vi "blokada wysylania manipulatora.vi"(6 "Y":i32, 8 "Zaxis":i32, 9 "X axis":i32, 10 "wysylanie":bool) -> (0 "zakres Z":bool, 1 "zakres X":bool, 2 "blokadaa":bool, 3 "Wyslij":bool, 4 "zakres Y":bool)   [LabVIEW 2015]
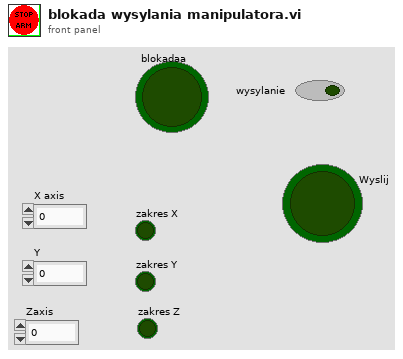
[diagram p1: front panel]
types:
  T1 = enum16{"Rising Edge", "Falling Edge", "Any Edge"}
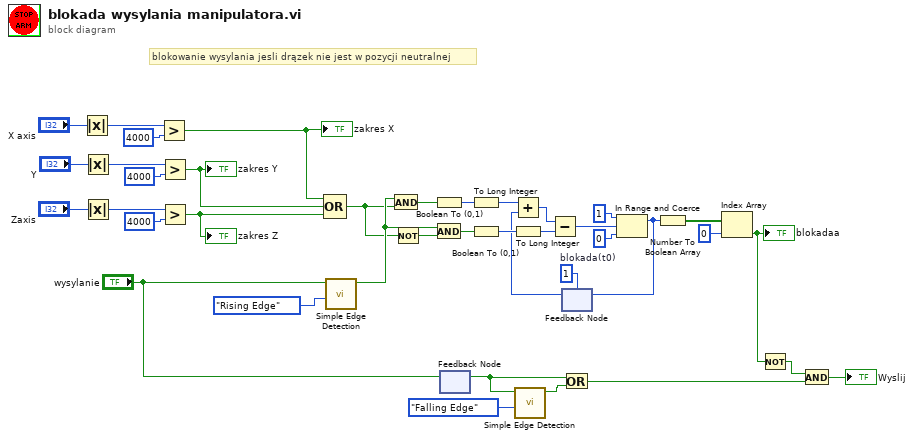
[diagram p0: block diagram]
diagram:
  w13 = 1  # blokada(t0)
  # "blokowanie wysylania jesli drązek nie jest w pozycji neutralnej"
  n1 = Absolute Value(x="X axis") -> (abs(x)=w23:i32)
  n2 = Absolute Value(x="Y") -> (abs(x)=w37:i32)
  n3 = Absolute Value(x="Zaxis") -> (abs(x)=w20:i32)
  n4 = Greater?(x=w23, y=4000) -> (0:w12:bool)
  "zakres X" <- w12
  n5 = Greater?(x=w37, y=4000) -> (0:w11:bool)
  "zakres Y" <- w11
  n6 = Greater?(x=w20, y=4000) -> (0:w10:bool)
  "zakres Z" <- w10
  n7 = Compound Arithmetic op=OR(w12, w11, w10) -> (w9:bool)
  n8 = call "Simple Edge Detection.vi"("Mode"=T1."Rising Edge", "clk_in"="wysylanie") -> ("edge?"=w31:bool)  [unwired: 9 in]
  n9 = And(x=w31, y=w9) -> (x .and. y?=w26:bool)
  n10 = Not(x=w9) -> (.not. x?=w30:bool)
  n11 = Boolean To (0,1)(Boolean=w26) -> (0, 1=w18:i16)
  n12 = And(x=w31, y=w30) -> (x .and. y?=w29:bool)
  n13 = feedback #1() -> (w4:bool)  [unwired: 1 in]
  n14 = feedback-in #1("wysylanie") -> ()
  n15 = To Long Integer(number=w18) -> (32bit integer=w19:i32)
  n16 = Boolean To (0,1)(Boolean=w29) -> (0, 1=w16:i16)
  n17 = To Long Integer(number=w16) -> (32bit integer=w17:i32)
  n18 = call "Simple Edge Detection.vi"("Mode"=T1."Falling Edge", "clk_in"=w4) -> ("edge?"=w3:bool)  [unwired: 9 in]
  n19 = feedback #2(w13) -> (w15:i32)
  n20 = Add(x=w19, y=w15) -> (x+y=w33:i32)
  n21 = Subtract(x=w33, y=w17) -> (x-y=w32:i32)
  n22 = Or(x=w4, y=w3) -> (x .or. y?=w2:bool)
  n23 = In Range and Coerce(upper limit=1 ("lower limit"), x=w32, lower limit=0) -> (coerced(x)=w14:i32)  [unwired: 1 out]
  n24 = feedback-in #2(w14) -> ()
  n25 = Number To Boolean Array(number=w14) -> (Boolean array=w34:bool[])
  n26 = Index Array(array=w34, index=0) -> (element=w1:bool)
  "blokadaa" <- w1
  n27 = Not(x=w1) -> (.not. x?=w7:bool)
  n28 = And(x=w7, y=w2) -> (x .and. y?=→"Wyslij":bool)
